vi "rsa_cryptor.vi"(1 "Modulo":string, 2 "Public exponent":string, 3 "Plaintext":string="HALLO") -> (0 "Encrypted text":string="HALLO")   [LabVIEW 2017]
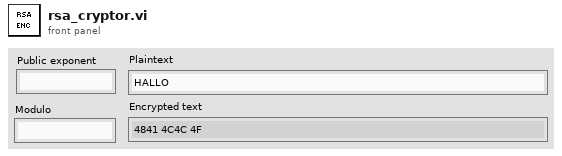
[diagram p1: front panel]
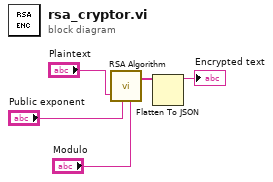
[diagram p0: block diagram]
diagram:
  n1 = call "RSA Algorithm.vi"("Plaintext"="Plaintext", "Exponent"="Public exponent", "Modulo"="Modulo") -> ("Output"=w2:string[])  [unwired: 3 in, 1 out]
  n2 = Flatten To JSON(anything=w2) -> (JSON string=→"Encrypted text":string)  [unwired: 2 in, 1 out]
